vi "Override Error.vi"(10 "Error":errorcluster, 11 "jettl Msg Override Error in":refnum<class "jettl Msg Override Error.lvclass">) -> (3 "jettl Msg Override Error out":refnum<class "jettl Msg Override Error.lvclass">)   [LabVIEW 2021, in "jettl Msg Override Error.lvlib" / "jettl Msg Override Error.lvclass"]
uses:
  jettl Msg Override Error.lvclass
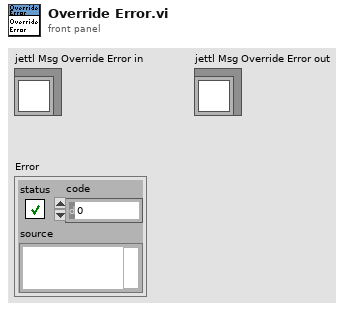
[diagram p1: front panel]
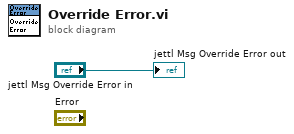
[diagram p0: block diagram]
diagram:
  "jettl Msg Override Error out" <- "jettl Msg Override Error in"
